vi "case structure.vi"() -> ()   [LabVIEW 2020]
panel:
  out "c":dbl
  in  "b":dbl
  in  "a":dbl
  in  "Opcion":i32
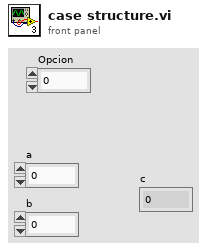
[diagram p1: front panel]
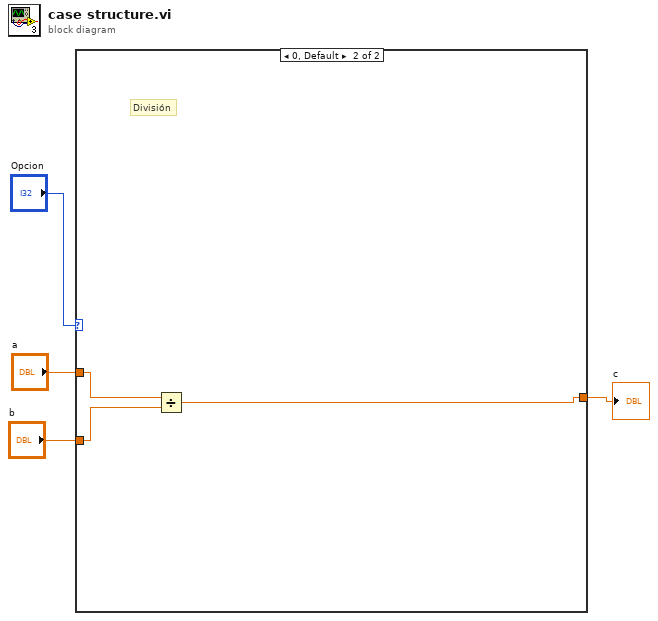
[diagram p0: block diagram]
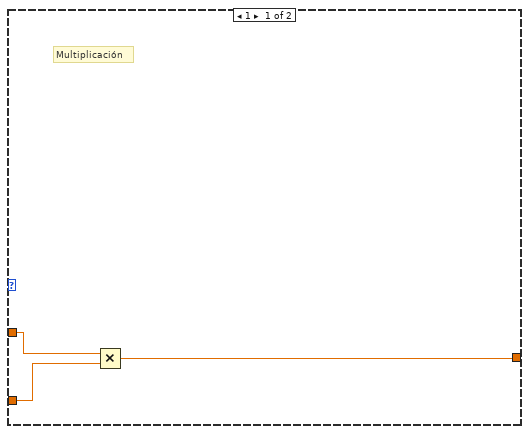
[diagram p2: hidden frame]
diagram:
  n1 = case shown="0, Default" "Opcion" {
    tunnel: "a" -> [w7 w10]
    tunnel: "b" -> [w6 w9]
    tunnel: [w5 w8] -> w1
    frame 1 {
      # "Multiplicación"
      n2 = Multiply(x=w7, y=w6) -> (x*y=w5:dbl)
    }
    frame 0, Default {
      # "División"
      n3 = Divide(x=w10, y=w9) -> (x/y=w8:dbl)
    }
  }
  "c" <- w1
